vi "Call Function with Python Object Return.vi"(8 "error in (no error)":errorcluster) -> (0 "error out":errorcluster)   [LabVIEW 2020]
uses:
  G-Embedded-Python-Interpreter-Toolkit/Merge Call Library Errors.vi
  <vilib>/addons/_JKI Toolkits/Caraya/classes/Assert/Assert Equal Value and Type_Variant.vi
  G-Embedded-Python-Interpreter-Toolkit/G-Embedded-Python-Interpreter-Toolkit.lvlib
  <vilib>/addons/_JKI Toolkits/Caraya/classes/Test/Test.lvclass
  <vilib>/addons/_JKI Toolkits/Caraya/classes/Assert/Assert.lvclass
panel:
  out "Value":i32
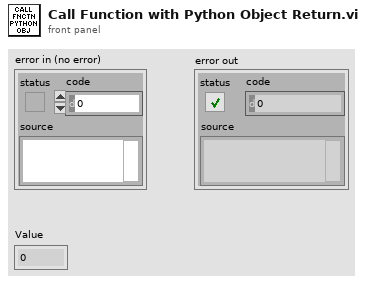
[diagram p1: front panel]
types:
  T1 = typedef "G-Embedded-Python-Interpreter-Toolkit.lvlib/Python Object Reference.ctl" = refnum<k1>
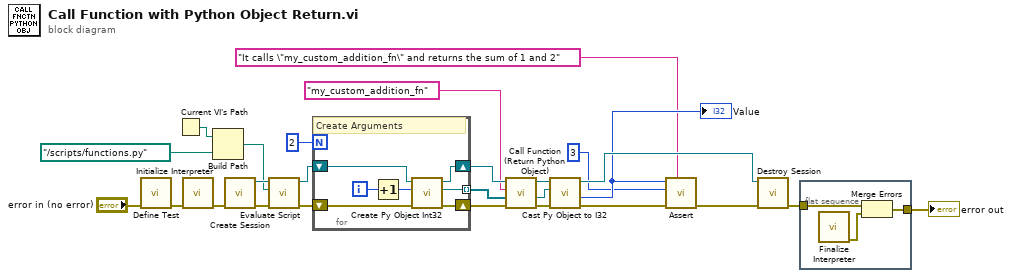
[diagram p0: block diagram]
diagram:
  n1 = call <vilib>:"Define Test.vi"("error in (no error)"="error in (no error)") -> ("error out"=w26:errorcluster)  [unwired: 10 in]
  n2 = Current VI's Path() -> (path=w21:path)
  n3 = call "Initialize Interpreter.vi"("error in (no error)"=w26) -> ("error out"=w23:errorcluster)  [unwired: 9 in, 1 out]
  n4 = Build Path(base path=w21, name or relative path=path "../scripts/functions.py" ("Path")) -> (appended path=w19:path)
  n5 = call "Create Session.vi"("error in (no error)"=w23) -> ("error out"=w18:errorcluster, "Session Handle"=w22:refnum<data-value>)  [unwired: 9 in]
  n6 = call "Evaluate Script.vi"("error in (no error)"=w18, "Script File Path"=w19, "Session Handle in"=w22) -> ("error out"=w15:errorcluster, "Session Handle out"=w16:refnum<data-value>)  [unwired: 7 in]
  n7 = for {
    N: 2 -> [_]
    shift-right: [w29] -> w13
    shift-left: w16 -> [w33]
    shift-right: [w30] -> w14
    shift-left: w15 -> [w32]
    tunnel: [w28] -> w11 mode=indexing
    i -> [w31]
    # "Create Arguments"
    n8 = Increment(x=w31) -> (x+1=w27:i32)
    n9 = call "Create Py Object Int32.vi"("error in (no error)"=w32, "Value"=w27, "Session Handle in"=w33) -> ("error out"=w30:errorcluster, "Python Object Refnum"=w28:T1, "Session Handle out"=w29:refnum<data-value>)  [unwired: 6 in]
  }
  n10 = call "Call Function (Return Python Object).vi"("error in (no error)"=w14, "Arguments"=w11, "Function Name"="my_custom_addition_fn", "Session Handle in"=w13) -> ("error out"=w8:errorcluster, "Returned Python Object Refnum"=w9:T1, "Session Handle out"=w10:refnum<data-value>)  [unwired: 5 in]
  n11 = call "Cast Py Object to I32.vi"("error in (no error)"=w8, "Python Object Refnum in"=w9, "Session Handle in"=w10) -> ("error out"=w4:errorcluster, "Value"=w5:i32, "Session Handle out"=w7:refnum<data-value>)  [unwired: 5 in, 1 out]
  "Value" <- w5
  n12 = call-poly <vilib>:"Assert.vi"("Label"="It calls \"my_custom_addition_fn\" and returns the sum of 1 and 2", "error in (no error)"=w4, "Y"=3 ("Value"), "X"=w5) -> ("error out"=w3:errorcluster)  [unwired: 7 in]
  n13 = call "Destroy Session.vi"("error in (no error)"=w3, "Session Handle"=w7) -> ("error out"=w17:errorcluster)  [unwired: 9 in]
  n14 = flat-sequence {
    tunnel: w17 -> [w36]
    tunnel: [w34] -> w24
    frame #0 {
      n15 = call "Finalize Interpreter.vi"() -> ("error out"=w35:errorcluster)  [unwired: 11 in]
      n16 = Merge Errors(w36, w35) -> (w34:errorcluster)
    }
  }
  "error out" <- w24
